vi "FetchMultiPoint.vi"(8 "error in (no error)":errorcluster, 11 "HP3458aDMM in":refnum<class "HP3458aDMM.lvclass">) -> (0 "error out":errorcluster, 3 "HP3458aDMM out":refnum<class "HP3458aDMM.lvclass">)   [LabVIEW 2014, in "SamplerPlugins.lvlib" / "HP3458aDMM.lvclass"]
uses:
  HP3458aDMM.lvclass
  NISTSamplerPluginsBaseClass/TypeDefs/MultiPointReadingParams.ctl
  NISTSamplerPluginsBaseClass/SamplerPluginsBase.lvclass
  <instrlib>/Agilent 3458/Agilent 3458.lvlib
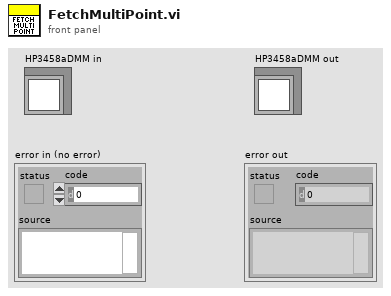
[diagram p1: front panel]
types:
  T1 = enum16{"ASCII", "Single Real", "Double Real", "Single Integer", "Double Integer"}
  T2 = typedef "SamplerPlugins.lvlib/SamplerPluginsBase.lvclass/MultiPointReadingParams.ctl" = cluster{"dReadingArray":dbl[], "iActualPts":i32, "Timestamp":dbl}
  T3 = typedef "SamplerPlugins.lvlib/SamplerPluginsBase.lvclass/ReadMultiPointParams.ctl" = cluster{"iMaxTimeMilliseconds":i32, "iArraySize":i32}
  T4 = typedef "SamplerPlugins.lvlib/SamplerPluginsBase.lvclass/ConfigMultiPointParams.ctl" = cluster{"iTriggerCount":i32, "iSampleCount":i32, "eSampleClock":u16, "dSampleInterval":dbl}
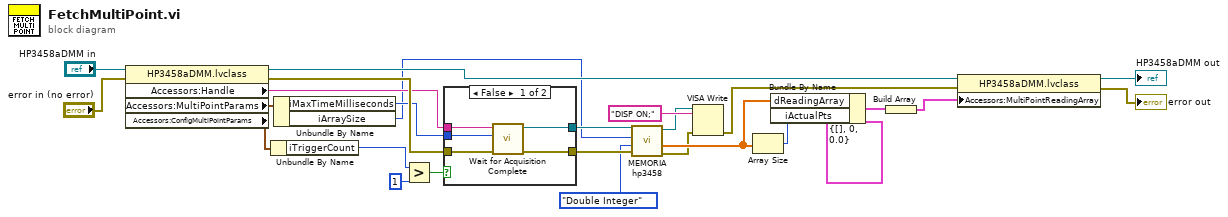
[diagram p0: block diagram]
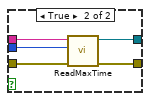
[diagram p2: hidden frame]
diagram:
  n1 = property class="HP3458aDMM.lvclass"(reference="HP3458aDMM in", error in="error in (no error)") -> (reference out=w21:refnum<class "HP3458aDMM.lvclass">, error out=w15:errorcluster, "Accessors:Handle"=w13:string, "Accessors:MultiPointParams"=w25:T3, "Accessors:ConfigMultiPointParams"=w19:T4)
  n2 = Unbundle By Name(w19) -> ("iTriggerCount"=w17:i32)
  n3 = Unbundle By Name(w25) -> ("iMaxTimeMilliseconds"=w14:i32, "iArraySize"=w9:i32)
  n4 = Greater?(x=w17, y=1) -> (0:w16:bool)
  n5 = case shown="False" w16 {
    tunnel: w15 -> [w29 w36]
    tunnel: w14 -> [w30 w35]
    tunnel: w13 -> [w31 w34]
    tunnel: [w28 w33] -> w12
    tunnel: [w27 w32] -> w11
    frame False {
      n6 = call <instrlib>:"Wait for Acquisition Complete.vi"("error in (no error)"=w29, "Maximum Time (10000 ms)"=w30, "VISA resource name"=w31) -> ("error out"=w28:errorcluster, "VISA resource name out"=w27:refnum<visa-resource-name>)  [unwired: 7 in]
    }
    frame True {
      n7 = call "ReadMaxTime.vi"("error in (no error)"=w36, "iMaxTimeMilliseconds"=w35, "HandleIn"=w34) -> ("error out"=w33:errorcluster, "HandleOut"=w32:refnum<visa-resource-name>)  [unwired: 7 in]
    }
  }
  n8 = call "MEMORIA hp3458.vi"("error in (no error)"=w12, "Output Format (0:ASCII)"=T1."Double Integer", "Número de muestras totales"=w9, "VISA session"=w11) -> ("error out"=w6:errorcluster, "Muestras digitales"=w7:dbl[], "dup VISA session"=w4:refnum<visa-resource-name>)  [unwired: 4 in, 1 out]
  n9 = VISA Write(VISA resource name=w4, write buffer="DISP ON;", error in (no error)=w6) -> (error out=w3:errorcluster)  [unwired: 2 out]
  n10 = Array Size(array=w7) -> (size(s)=w8:i32)
  n11 = Bundle By Name(cluster=T2 {"dReadingArray"=[], "iActualPts"=0, "Timestamp"=0.0} ("MultiPointReadingParams"), "dReadingArray"=w7, "iActualPts"=w8) -> (w2:T2)
  n12 = Build Array(w2) -> (w1:T2[])
  n13 = property class="HP3458aDMM.lvclass"(reference=w21, error in=w3, "Accessors:MultiPointReadingArray"=w1) -> (reference out=→"HP3458aDMM out":refnum<class "HP3458aDMM.lvclass">, error out=→"error out":errorcluster)
